vi "SRV_Parse IMJ Data.vi"(0 "##IMJ Data":string) -> (6 "frame size in pixels":string, 8 "Frame Size in Bytes":u32, 10 "Rest of frame data":string)   [LabVIEW 2009]
doc: "<B>x = frame size in pixels:</B>\n1 = 80x64\n3 = 160x120\n5 = 320x240\n7 = 640x480\n9 = 1280x1024"
uses:
  <vilib>/Utility/error.llb/whitespace.ctl
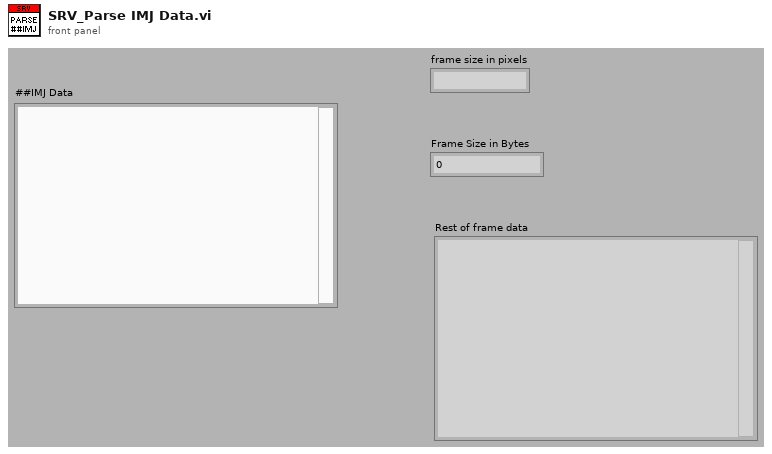
[diagram p1: front panel]
types:
  T1 = typedef "whitespace.ctl" = u16
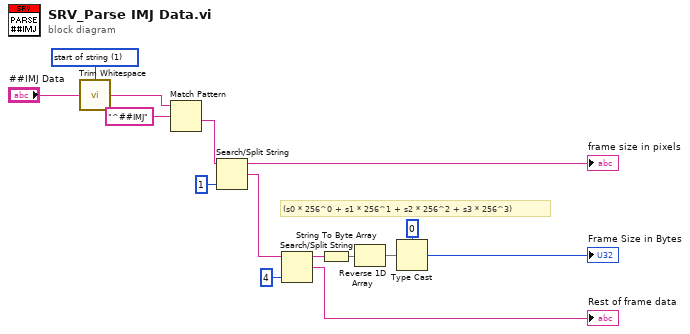
[diagram p0: block diagram]
diagram:
  w14 = T1 1 items=["both", "start of string", "end of string"] ("location (both)")
  # "(s0 * 256^0 + s1 * 256^1 + s2 * 256^2 + s3 * 256^3)"
  n1 = call <vilib>:"Trim Whitespace.vi"("string"="##IMJ Data", "location (both)"=w14) -> ("trimmed string"=w13:string)
  n2 = Match Pattern(string=w13, regular expression="^##IMJ") -> (after substring=w11:string)  [unwired: 1 in, 3 out]
  n3 = Search/Split String(string=w11, offset (0)=1) -> (substring before match=→"frame size in pixels":string, match + rest of string=w7:string)  [unwired: 1 in, 1 out]
  n4 = Search/Split String(string=w7, offset (0)=4) -> (substring before match=w3:string, match + rest of string=→"Rest of frame data":string)  [unwired: 1 in, 1 out]
  n5 = String To Byte Array(string=w3) -> (unsigned byte array=w6:u8[])
  n6 = Reverse 1D Array(array=w6) -> (reversed array=w4:u8[])
  n7 = Type Cast(type=u32 0 ("offset (0)"), x=w4) -> (*(type *) &x=→"Frame Size in Bytes":u32)
